vi "_NameCacher.vi"(10 "key":string, 11 "cacher":variant) -> (1 "Raw name":string, 2 "Key in lower case":string, 3 "cacher out":variant)   [LabVIEW 2017, in "TagDB.lvlib"]
uses:
  TagDB.lvlib
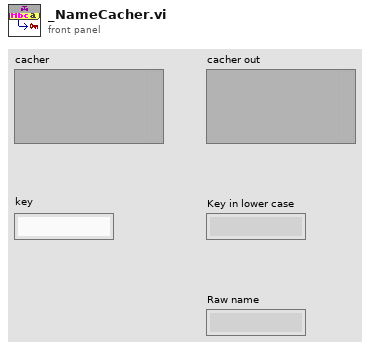
[diagram p1: front panel]
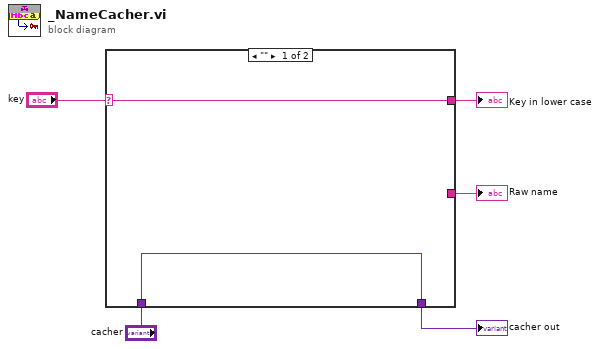
[diagram p0: block diagram]
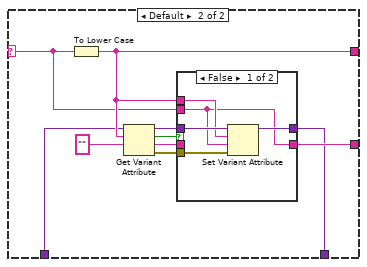
[diagram p2: hidden frame]
diagram:
  n1 = case shown="\"\"" "key" {
    selector: "key" -> [w7 w13]
    tunnel: [w7 w16] -> w5
    tunnel: [_ w10] -> w3
    tunnel: "cacher" -> [w6 w9]
    tunnel: [w6 w8] -> w2
    frame "" {
    }
    frame Default {
      n2 = To Lower Case(string=w13) -> (all lower case string=w16:string)
      n3 = Get Variant Attribute(Variant=w9, name=w16, default value (empty Variant)="") -> (duplicate Variant=w17:variant, found=w14:bool, value=w12:string, error out=w11:errorcluster)  [unwired: 1 in]
      n4 = case shown="False" w14 {
        tunnel: w17 -> [w22 w24]
        tunnel: w16 -> [w21 _]
        tunnel: w13 -> [w18 _]
        tunnel: w12 -> [_ w23]
        tunnel: w11 -> [w20 _]
        tunnel: [w19 w24] -> w8
        tunnel: [w18 w23] -> w10
        frame False {
          n5 = Set Variant Attribute(Variant=w22, name=w21, value=w18, error in=w20) -> (Variant out=w19:variant)  [unwired: 2 out]
        }
        frame True {
        }
      }
    }
  }
  "Key in lower case" <- w5
  "Raw name" <- w3
  "cacher out" <- w2
